vi "Decompress.vi"(8 "error in (no error)":errorcluster, 10 "compressed data":string) -> (0 "error out":errorcluster, 2 "uncompressed data":string)   [LabVIEW 2020, in "lvzstd.lvlib"]
uses:
  lvzstd.lvlib
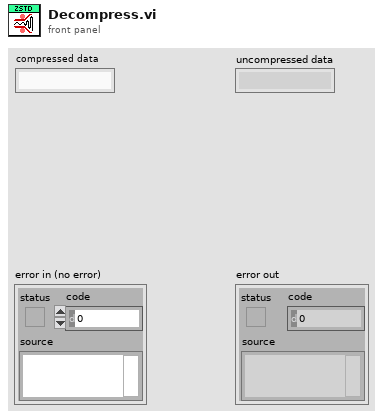
[diagram p1: front panel]
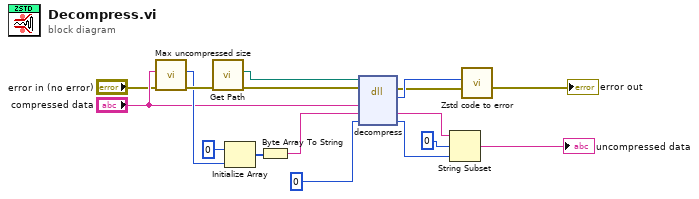
[diagram p0: block diagram]
diagram:
  n1 = call "Max uncompressed size.vi"("error in (no error)"="error in (no error)", "srcHandle"="compressed data") -> ("error out"=w5:errorcluster, "uncompressed size"=w4:i32)  [unwired: 8 in]
  n2 = call "Get Path.vi"("error in (no error)"=w5) -> ("error out (no error)"=w6:errorcluster, "Library Path"=w1:path)  [unwired: 9 in]
  n3 = Initialize Array(u8 0, w4) -> (w16:u8[])
  n4 = Byte Array To String(unsigned byte array=w16) -> (string=w15:string)
  n5 = dll-call lib="?" fn="decompress"(path in=w1, error in=w6, "srcHandle"="compressed data", "dstHandle"=w15, "uncompressedSize"=0 ("compressedSize")) -> (error out=w8:errorcluster, "return type"=w13:i32, "dstHandle"=w12:string, "uncompressedSize"=w11:i32)  [unwired: 2 in, 1 out]
  n6 = String Subset(string=w12, offset (0)=0, length (rest)=w11) -> (substring=→"uncompressed data":string)
  n7 = call "Zstd code to error.vi"("error in"=w8, "Error code"=w13) -> ("error in (no error)"=→"error out":errorcluster)  [unwired: 9 in]
